vi "Read Configuration Interface.vi"(11 "Configuration Interface Test In":refnum<class "Configuration Interface Test.lvclass">) -> (2 "Configuration":refnum<class "Configuration.lvclass">, 3 "Configuration Interface Test Out":refnum<class "Configuration Interface Test.lvclass">)   [LabVIEW 2020, in "Configuration Interface Test.lvclass"]
uses:
  Configuration Interface Test.lvclass
  source/Framework/Configuration/Configuration.lvclass
  Configuration Interface Test.lvclass/Configuration Interface Test.ctl
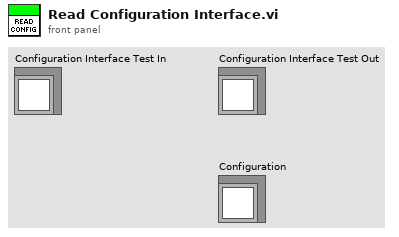
[diagram p1: front panel]
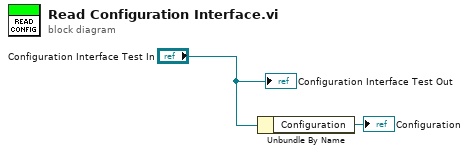
[diagram p0: block diagram]
diagram:
  n1 = Unbundle By Name("Configuration Interface Test In") -> ("Configuration"=→"Configuration":refnum<class "Configuration.lvclass">)
  "Configuration Interface Test Out" <- "Configuration Interface Test In"
